vi "calc_alpha_beta.vi"(3 "Frequency (GHz)":dbl) -> (0 "Beta":dbl, 1 "Alpha":dbl)   [LabVIEW 2015]
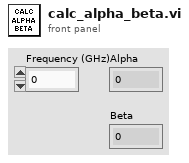
[diagram p1: front panel]
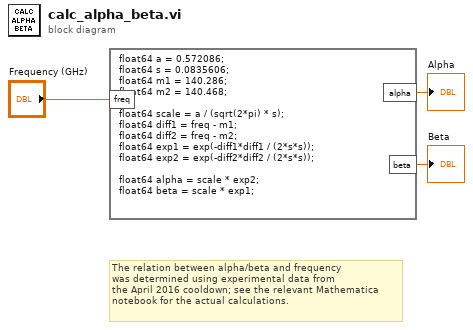
[diagram p0: block diagram]
diagram:
  # "The relation between alpha/beta and frequency\nwas determined using experimental data from\nthe April 2016 cooldown; see the relevant Mathematica\nnotebook for the actual calculations."
  n1 = formula code="float64 a = 0.572086;\nfloat64 s = 0.0835606;\nfloat64 m1 = 140.286;\nfloat64 m2 = 140.468;\n\nfloat64 scale = a / (sqrt(2*pi) * s);\nfloat64 diff1 = freq - m1;\nfloat64 diff2 = freq - m2;\nfloat64 exp1 = exp(-diff1*diff1 / (2*s*s));\nfloat64 exp2 = exp(-diff2*diff2 / (2*s*s));\n\nfloat64 alpha = scale * exp2;\nfloat64 beta = scale * exp1;"("freq"="Frequency (GHz)") -> ("alpha"=→"Alpha":dbl, "beta"=→"Beta":dbl)
